vi "_UtilsRandomBoolArray.vi"(1 "array size":i32=256, 2 "factor":dbl=1.0) -> (0 "array":bool[](array[boolean]))   [LabVIEW 2014, in "examples.lvlib"]
uses:
  examples.lvlib
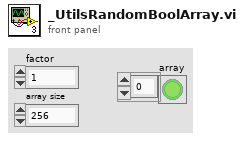
[diagram p1: front panel]
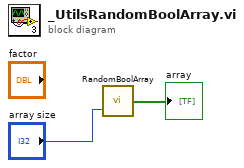
[diagram p0: block diagram]
diagram:
  n1 = call "RandomBoolArray.vi"("random array size"="array size") -> ("random array"=→"array":bool[])  [unwired: 1 in]
